vi "temp To HTML Improovd.vi"(0 "temperatuur 3":refnum<vi>, 1 "path to JPEG file":path) -> ()   [LabVIEW 2013]
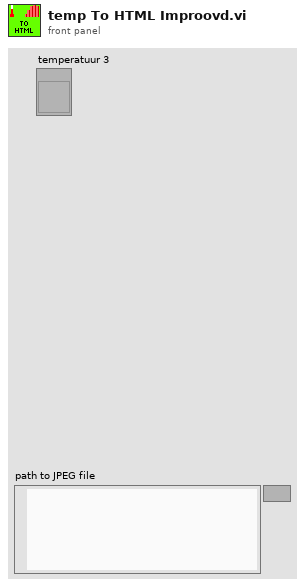
[diagram p1: front panel]
types:
  T1 = typedef "imagedata.ctl" = cluster{"image type":i32, "image depth":i32, "image":u8[], "mask":u8[], "colors":u32[], "Rectangle":cluster{"left":i16, "top":i16, "right":i16, "bottom":i16}}
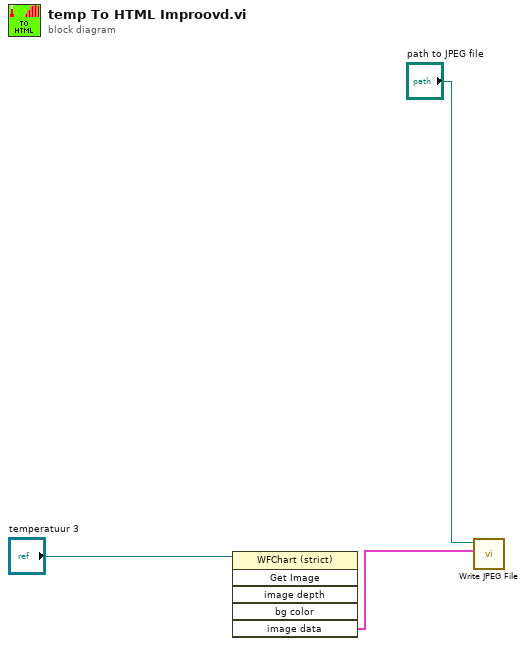
[diagram p0: block diagram]
diagram:
  n1 = invoke on="Invoke Node" class="WFChart (strict)" method="Get Image"(reference="temperatuur 3") -> ("image data"=w2:T1)  [unwired: 5 in, 5 out]
  n2 = call <vilib>:"Write JPEG File.vi"("image data"=w2, "path to JPEG file"="path to JPEG file") -> ()  [unwired: 8 in, 2 out]
